vi "Tank Fill Global.vi"() -> ()   [LabVIEW 2013]
panel:
  out "Tank level":i32
  out "Bottom":bool
  out "Top":bool
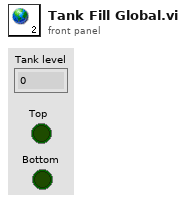
[diagram p1: front panel]
diagram:
